vi "Add User Defined Group.vi"(8 "error in (no error)":errorcluster, 11 "Node Ptr":u64 format="%.0x") -> (0 "error out":errorcluster)   [LabVIEW 2019, in "Diagnostics Addon System Explorer.lvlib"]
uses:
  Diagnostics Addon System Explorer.lvlib
  Addon Shared/SubVIs/Constants.vi
  Addon Shared/Diagnostics Addon Shared.lvlib
  <vilib>/NI VeriStand/Custom Device API/Custom Device API.lvlib
  <vilib>/NI/NI VeriStand Advanced SysDef API/SysDef API/Advanced System Definition.lvlib
panel:
  in  "Tag":string
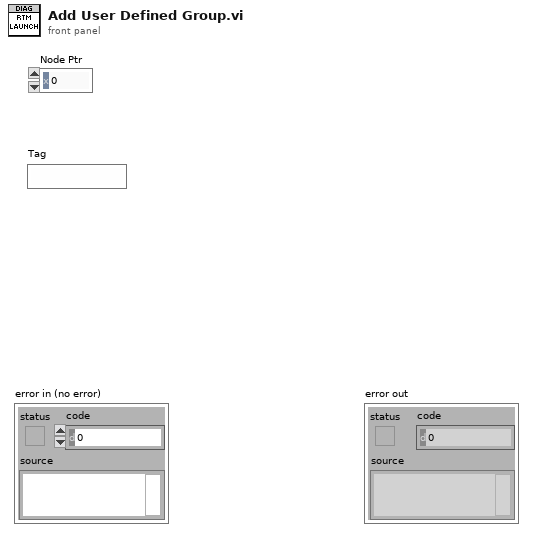
[diagram p1: front panel]
types:
  T1 = typedef "Custom Device API.lvlib/Custom Device Item Ref.ctl" = u64
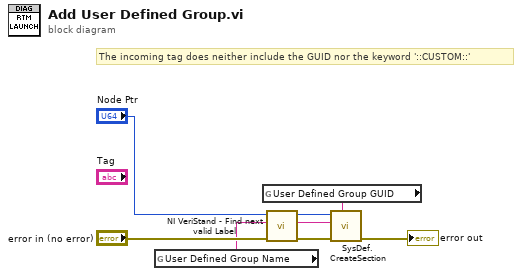
[diagram p0: block diagram]
diagram:
  # "The incoming tag does neither include the GUID nor the keyword '::CUSTOM::'"
  n1 = global read "Constants.vi" "User Defined Group Name"() -> (w1:string)
  n2 = global read "Constants.vi" "User Defined Group GUID"() -> (w8:string)
  n3 = call <vilib>:"NI VeriStand - Find next valid Label.vi"("error in (no error)"="error in (no error)", "Label"=w1, "Item Ref in"="Node Ptr") -> ("error out"=w6:errorcluster, "Label out"=w5:string, "Item Ref out"=w7:T1)  [unwired: 4 in, 2 out]
  n4 = call <vilib>:"SysDef.CreateSection.vi"("GUID"=w8, "error in (no error)"=w6, "Name"=w5, "nodeID"=w7) -> ("error out"=→"error out":errorcluster)  [unwired: 4 in, 3 out]
